vi "KBRD Query Pan Position v2 (SubVI).vi"(11 "Queue in":refnum<queue>) -> (3 "queue out":refnum<queue>)   [LabVIEW 2018]
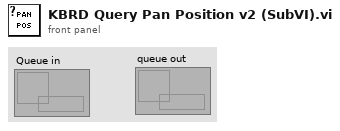
[diagram p1: front panel]
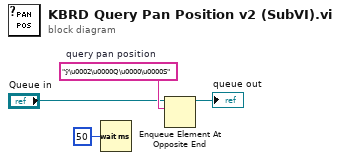
[diagram p0: block diagram]
diagram:
  w4 = "ÿ\u0002\u0000Q\u0000\u0000S"  # query pan position
  n1 = Wait (ms)(milliseconds to wait=u32 50) -> ()  [unwired: 1 out]
  n2 = Enqueue Element At Opposite End(queue="Queue in", element=w4) -> (queue out=→"queue out":refnum<queue>)  [unwired: 2 in, 2 out]
